vi "CASE STRUCTURE.vi"() -> ()   [LabVIEW 2017]
panel:
  out "Color Box":u32(colorbox)
  in  "Boolean":bool
  out "OUTPUT":dbl
  in  "B":dbl
  in  "A":dbl
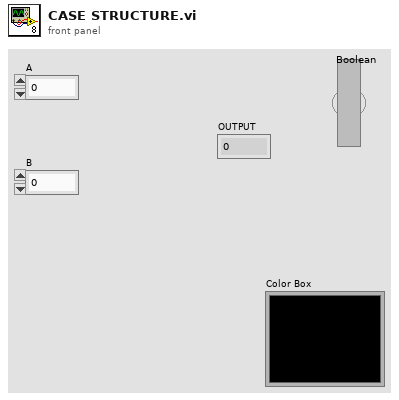
[diagram p1: front panel]
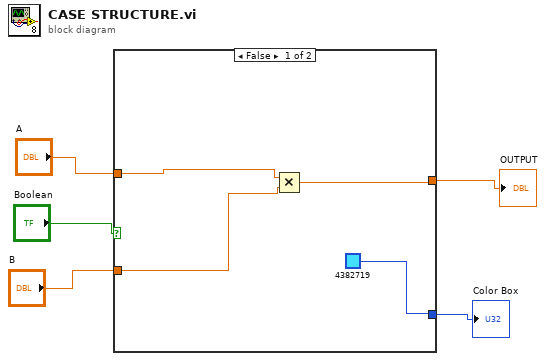
[diagram p0: block diagram]
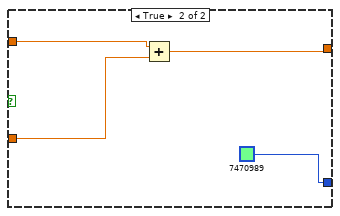
[diagram p2: hidden frame]
diagram:
  n1 = case shown="False" "Boolean" {
    tunnel: "A" -> [w8 w13]
    tunnel: "B" -> [w9 w12]
    tunnel: [w7 w11] -> w2
    tunnel: [u32 4382719 u32 7470989] -> w1
    frame False {
      n2 = Multiply(x=w8, y=w9) -> (x*y=w7:dbl)
    }
    frame True {
      n3 = Add(x=w13, y=w12) -> (x+y=w11:dbl)
    }
  }
  "OUTPUT" <- w2
  "Color Box" <- w1
